vi "SetRegister.vi"(3 "Data":u32, 4 "Offset":u32=8, 5 "error in (no error)":errorcluster) -> (0 "error out":errorcluster)   [LabVIEW 2015]
uses:
  BC637PCI.dll
panel:
  out "Data":string
  out "Offset":string
  out "Return":i32
  # "Decimal"
  # "Hexidecimal"
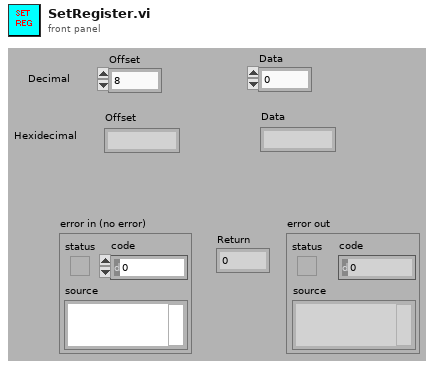
[diagram p1: front panel]
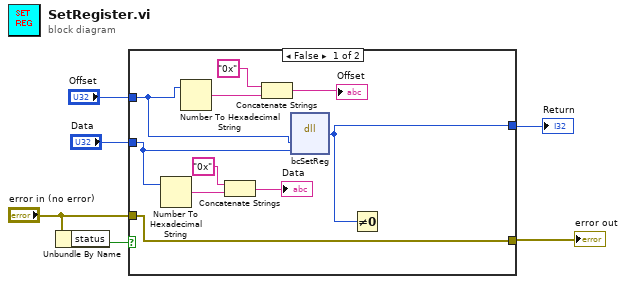
[diagram p0: block diagram]
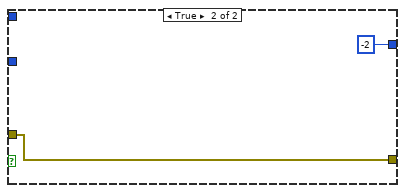
[diagram p2: hidden frame]
diagram:
  n1 = Unbundle By Name("error in (no error)") -> ("status"=w5:bool)
  n2 = case shown="False" w5 {
    tunnel: [w7 w17] -> w6
    tunnel: "error in (no error)" -> [w7 w17]
    tunnel: [w16 -2] -> w3
    tunnel: "Data" -> [w14 _]
    tunnel: "Offset" -> [w15 _]
    frame False {
      n3 = Number To Hexadecimal String(2:w14) -> (0:w13:string)  [unwired: 1 in]
      n4 = Number To Hexadecimal String(2:w15) -> (0:w10:string)  [unwired: 1 in]
      n5 = Concatenate Strings("0x", w13) -> (→"Data":string)
      n6 = Concatenate Strings("0x", w10) -> (→"Offset":string)
      n7 = dll-call lib="C:/ALPHA GSCS/GSCS/Systems/SIcamera_Control/GPS_Drivers/BC637PCI.dll" fn="bcSetReg"("offset"=w15, "data"=w14) -> ("return type"=w16:i32)  [unwired: 5 in, 2 out]
      n8 = Not Equal To 0?(x=w16) -> ()  [unwired: 1 out]
    }
    frame True {
    }
  }
  "error out" <- w6
  "Return" <- w3
